vi "stations configure instrument.vi"(8 "error in (no error)":errorcluster, 9 "port number (3363)":u16=3363, 11 "POST (empty)":T1) -> (0 "error out":errorcluster, 2 "Serial Number":string, 3 "Configuration":string, 4 "LastCal":dbl, 6 "CalDue":dbl)   [LabVIEW 2011]
uses:
  Addons/internet/utils/keyedarr.llb/Keyed Array.ctl
  Addons/internet/utils/strutil.llb/Case Matching.ctl
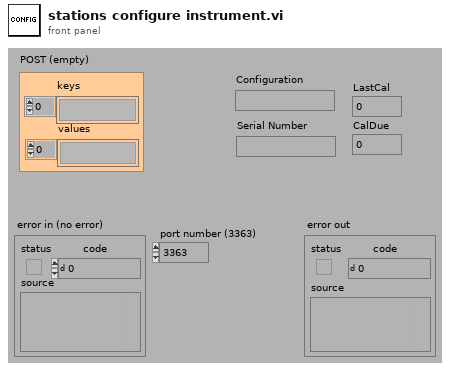
[diagram p1: front panel]
types:
  T1 = typedef "Keyed Array.ctl" = cluster{"keys":string[], "values":string[]}
  T2 = typedef "Case Matching.ctl" = enum16{"a != A", "a == A", "system"}
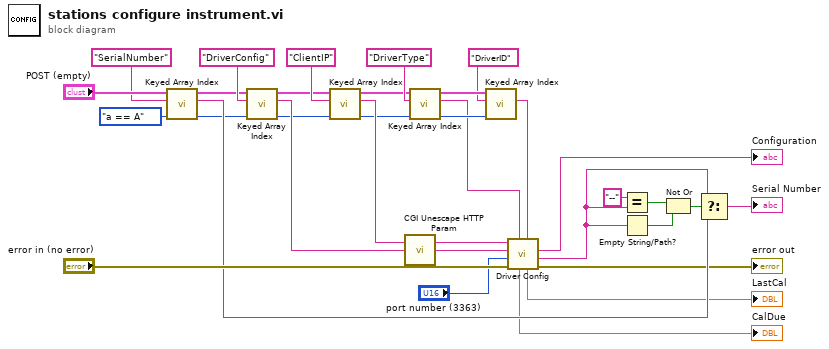
[diagram p0: block diagram]
diagram:
  w12 = Case_Matching."a == A" ("case matching (sensitive)")
  n1 = call "Keyed Array Index.vi"("case matching (sensitive)"=w12, "key"="SerialNumber" ("string"), "array in"="POST (empty)") -> ("value"=w25:string, "duplicate array"=w16:T1)  [unwired: 1 in, 2 out]
  n2 = call "Keyed Array Index.vi"("case matching (sensitive)"=w12, "key"="DriverConfig" ("string"), "array in"=w16) -> ("value"=w27:string, "duplicate array"=w15:T1)  [unwired: 1 in, 2 out]
  n3 = call "Keyed Array Index.vi"("case matching (sensitive)"=w12, "key"="ClientIP" ("string"), "array in"=w15) -> ("value"=w13:string, "duplicate array"=w14:T1)  [unwired: 1 in, 2 out]
  n4 = call "CGI Unescape HTTP Param.vi"("url-encoded string"=w27) -> ("string"=w5:string)
  n5 = call "Keyed Array Index.vi"("case matching (sensitive)"=w12, "key"="DriverType" ("string"), "array in"=w14) -> ("value"=w10:string, "duplicate array"=w24:T1)  [unwired: 1 in, 2 out]
  n6 = call "Keyed Array Index.vi"("case matching (sensitive)"=w12, "key"="DriverID" ("string"), "array in"=w24) -> ("value"=w11:string)  [unwired: 1 in, 3 out]
  n7 = call "Driver Config.vi"("DriverID (\"\")"=w11, "DriverType (\"\")"=w10, "error in (no error)"="error in (no error)", "port number (3363)"="port number (3363)", "Configuration In (Empty)"=w5, "TestStation Client (\"\")"=w13) -> ("error out"=→"error out":errorcluster, "Serial Number"=w4:string, "Configuration Out"=→"Configuration":string, "LastCal"=→"LastCal":dbl, "CalDue"=→"CalDue":dbl)  [unwired: 1 out]
  n8 = Equal?(x="--" ("y"), y=w4) -> (x = y?=w7:bool)
  n9 = Empty String/Path?(string/path=w4) -> (empty?=w8:bool)
  n10 = Not Or(1:w8, 2:w7) -> (0:w6:bool)
  n11 = Select(t=w4, s=w6, f=w25) -> (s? t:f=→"Serial Number":string)
